vi "ExtractScanPlane.vi"(5 "End Frame":i32, 6 "Header":T1, 7 "Start Frame":i32, 9 "Scan Plane":i32, 10 "PMT Channel":i32, 11 "All Scan Data":dbl[][][][](array[numeric])) -> (3 "Scan Plane Data":dbl[][][](array[numeric]))   [LabVIEW 2012]
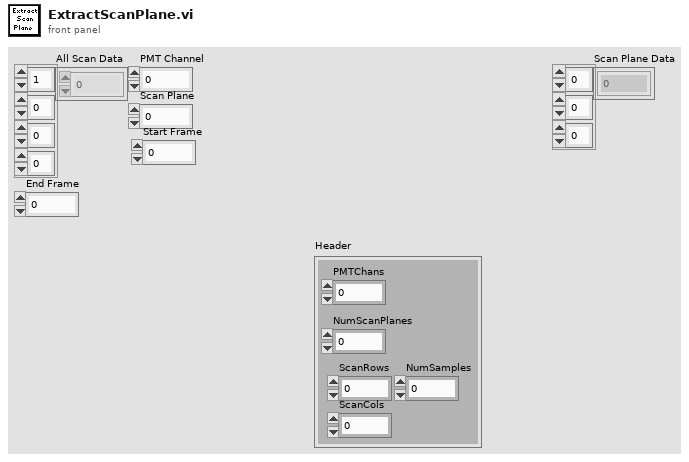
[diagram p1: front panel]
types:
  T1 = cluster{"PMTChans":i32, "NumScanPlanes":i32, "ScanRows":i32, "ScanCols":i32, "NumSamples":i32}
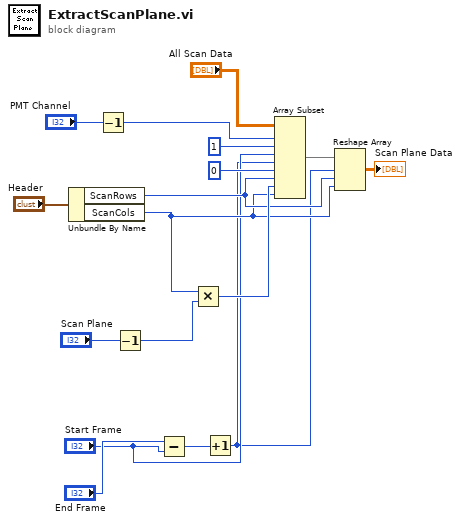
[diagram p0: block diagram]
diagram:
  n1 = Unbundle By Name("Header") -> ("ScanRows"=w7:i32, "ScanCols"=w6:i32)
  n2 = Decrement(x="PMT Channel") -> (x-1=w10:i32)
  n3 = Decrement(x="Scan Plane") -> (x-1=w13:i32)
  n4 = Subtract(x="End Frame", y="Start Frame") -> (x-y=w3:i32)
  n5 = Multiply(x=w6, y=w13) -> (x*y=w12:i32)
  n6 = Increment(x=w3) -> (x+1=w1:i32)
  n7 = Array Subset(array="All Scan Data", index (dim 0)=w10, length (dim 0)=1 ("length"), index (dim 1)="Start Frame", length (dim 1)=w1, index (dim 2)=0 ("index"), length (dim 2)=w7, index (dim 3)=w12, length (dim 3)=w6) -> (w17:dbl[][][][])
  n8 = Reshape Array(w17, w1, w7, w6) -> (→"Scan Plane Data":dbl[][][])
